vi "Actor Core.vi"(8 "error in":errorcluster, 11 "Nested in":refnum<class "ATM_UI_Controller.lvclass">) -> (0 "error out":errorcluster, 3 "Actor out":refnum<class "Actor.lvclass">)   [LabVIEW 2025, in "ATM_UI_Controller.lvlib" / "ATM_UI_Controller.lvclass"]
doc: "(<B>Filename</B>: Actor Framework.lvlib:Actor.lvclass:Actor Core.vi)\n\nReceives messages to the actor, reacts to them, and initiates any error handling that may shut the actor down.\n\nDescendant classes may override this VI to append parallel tasks for the actor to complete while it handles messages. Overrides use the Call Parent Method node."
uses:
  ATM_UI_Controller.lvclass
  <vilib>/ActorFramework/Actor/Actor.lvclass
  <vilib>/ActorFramework/Actor/Actor.lvclass/Actor.ctl
  <vilib>/ActorFramework/Message Enqueuer/Message Enqueuer.lvclass/Message Enqueuer.ctl
  ATM_UI_Controller.lvclass/ATM_UI_Controller.ctl
  <vilib>/ActorFramework/Message Enqueuer/Init from Existing Queue.vi
  <vilib>/ActorFramework/Message Enqueuer/Enqueue.vi
  <vilib>/ActorFramework/Stop Msg/Stop Msg.lvclass
  <vilib>/ActorFramework/Message Priority Queue/Priority Enqueue.vi
  <vilib>/ActorFramework/Message Enqueuer/Message Enqueuer.lvclass
  <vilib>/ni/Actors/State Actor/State Actor/State Actor.lvclass
  C:/Program Files (x86)/National Instruments/LabVIEW 2025/vi.lib/ni/Actors/State Actor/State Actor/State Actor.lvclass
  C:/Program Files (x86)/National Instruments/LabVIEW 2025/vi.lib/ActorFramework/Actor/Actor.lvclass
  C:/Users/halstead_rideriver/Documents/Labview_Practice/ATM_Machine_Actor Framework/ATM_ACTORFW/ATM_UI_Controller/ATM_UI_Controller.lvclass
panel:
  out "State-Status:":string
  in  "Start":bool
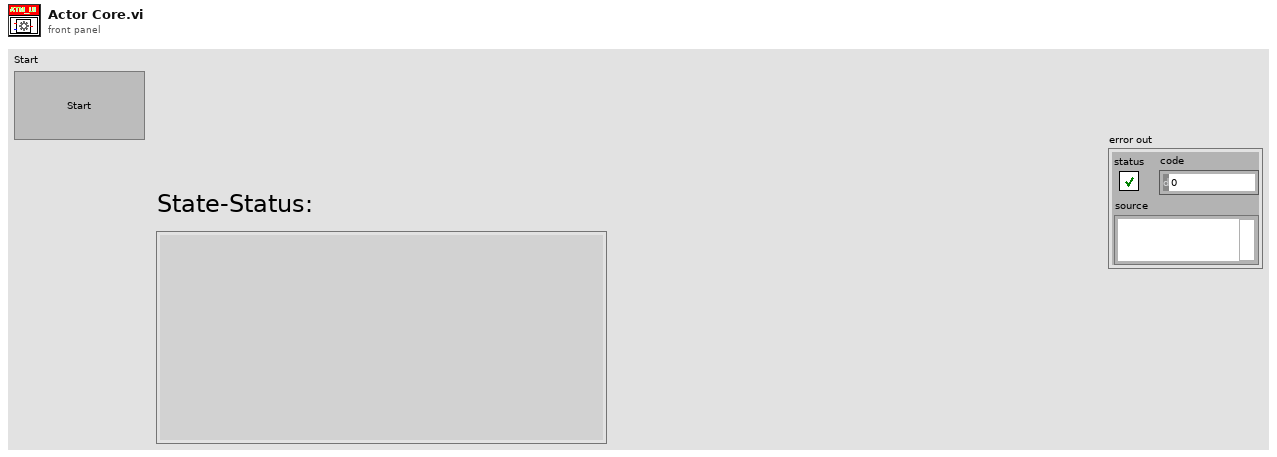
[diagram p1: front panel]
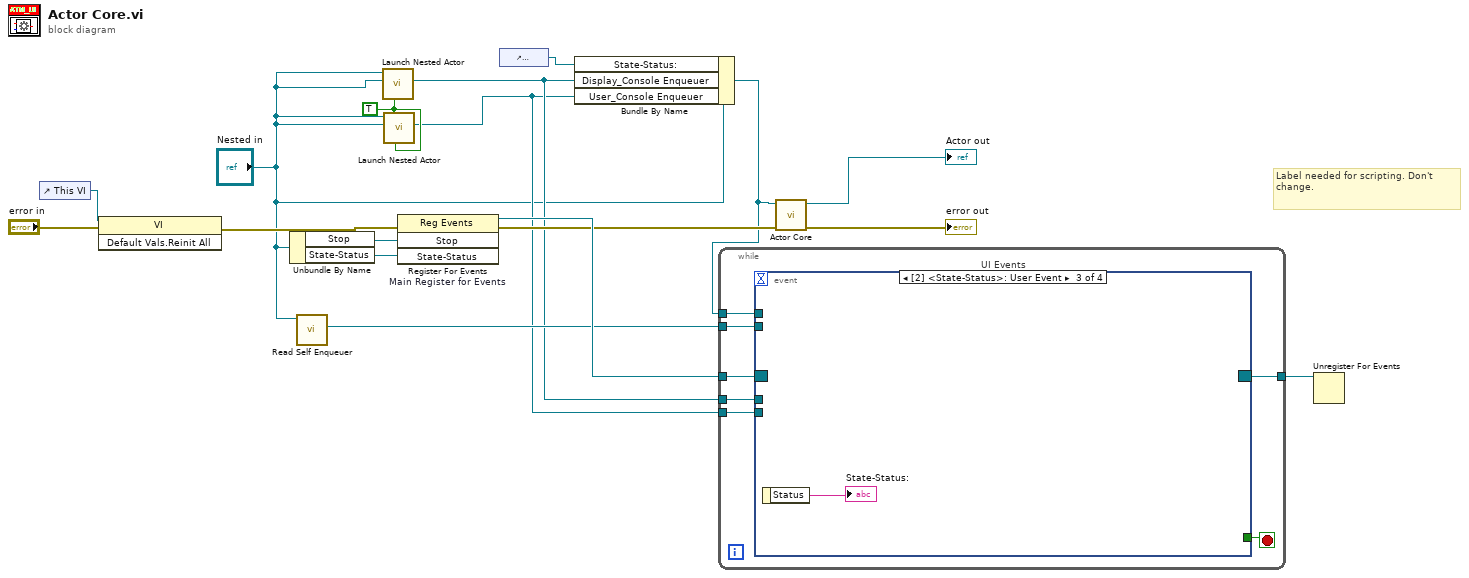
[diagram p0: block diagram]
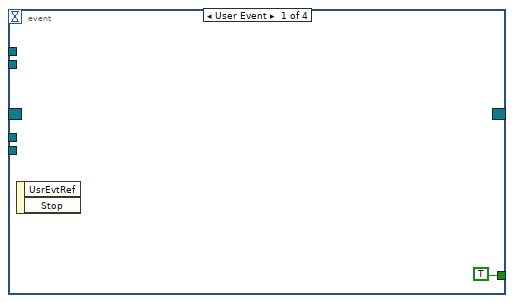
[diagram p2: hidden frame]
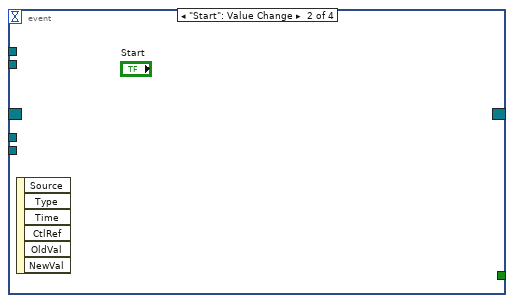
[diagram p3: hidden frame]
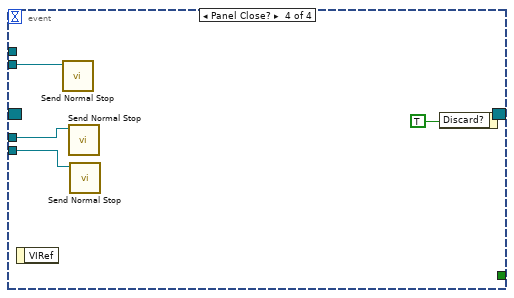
[diagram p4: hidden frame]
diagram:
  w9 = TRUE ("Open Actor Core front panel? (F)")
  # "Label needed for scripting. Don't change."
  n1 = control-ref of="This VI"() -> (w4:refnum<vi>)
  n2 = invoke class="VI" method="Default Vals.Reinit All"(reference=w4, error in="error in") -> (error out=w5:errorcluster)  [unwired: 1 in, 2 out]
  n3 = Unbundle By Name("Nested in") -> ("Stop"=w14:refnum<user-event>, "State-Status"=w1:refnum<user-event>)
  n4 = call <vilib>:"Read Self Enqueuer.vi"("Actor"="Nested in") -> ("Self Enqueuer"=w12:refnum<class "Message Enqueuer.lvclass">)  [unwired: 10 in]
  n5 = call <vilib>:"Launch Nested Actor.vi"("Open Actor Core front panel? (F)"=w9, "Nested Actor"="Nested in", "Caller Actor in"="Nested in") -> ("Nested Actor's Enqueuer"=w10:refnum<class "Message Enqueuer.lvclass">)  [unwired: 6 in, 2 out]
  n6 = call <vilib>:"Launch Nested Actor.vi"("Open Actor Core front panel? (F)"=w9, "Nested Actor"="Nested in", "Caller Actor in"="Nested in") -> ("Nested Actor's Enqueuer"=w8:refnum<class "Message Enqueuer.lvclass">)  [unwired: 6 in, 2 out]
  n7 = register-events "Main Register for Events"(error in=w5, w14, w1) -> (reference out=w15:refnum<event-registration>, error out=w11:errorcluster)  [unwired: 1 in]
  n8 = control-ref of="State-Status:"() -> (w2:refnum<vi>)
  n9 = Bundle By Name(cluster="Nested in", "State-Status:"=w2, "Display_Console Enqueuer"=w10, "User_Console Enqueuer"=w8) -> (w7:refnum<class "ATM_UI_Controller.lvclass">)
  n10 = while {
    tunnel: w15 -> [w24]
    tunnel: [w22] -> w13
    tunnel: w12 -> [w21]
    tunnel: w10 -> [w20]
    tunnel: w8 -> [w19]
    tunnel: w7 -> [w18]
    stop <- w23 stop-if-true
    n11 = event "UI Events" shown="[2] <State-Status>: User Event" {
      selector: w24 -> [_ _ _ _]
      dyn-events: [_ _ _ _] -> w22
      timeout: _ -> [_ _ _ _]
      tunnel: [TRUE _ _ _] -> w23
      tunnel: w21 -> [_ _ _ w29]
      tunnel: w20 -> [_ _ _ w28]
      tunnel: w19 -> [_ _ _ w27]
      tunnel: w18 -> [_ _ _ _]
      event User Event {
        n12 = event-data() -> ()  [unwired: 1 in, 2 out]
      }
      event "Start": Value Change {
        n13 = event-data() -> ()  [unwired: 1 in, 6 out]
      }
      event User Event {
        n14 = event-data() -> ("Status"=→"State-Status:":string)  [unwired: 1 in]
      }
      event Panel Close? {
        n15 = event-data() -> ()  [unwired: 1 in, 1 out]
        n16 = call <vilib>:"Send Normal Stop.vi"("Message Enqueuer"=w29) -> ()  [unwired: 10 in, 1 out]
        n17 = call <vilib>:"Send Normal Stop.vi"("Message Enqueuer"=w28) -> ()  [unwired: 10 in, 1 out]
        n18 = call <vilib>:"Send Normal Stop.vi"("Message Enqueuer"=w27) -> ()  [unwired: 10 in, 1 out]
        n19 = event-data("Discard?"=TRUE) -> ()  [unwired: 1 in, 1 out]
      }
    }
  }
  n20 = call-parent "Actor Core.vi"("error in"=w11, "State in"=w7) -> ("error out"=→"error out":errorcluster, "Actor out"=→"Actor out":refnum<class "Actor.lvclass">)  [unwired: 8 in]
  n21 = Unregister For Events(event registration refnum=w13) -> ()  [unwired: 1 in, 1 out]
